vi "Parse PJVS Voltages.vi"(8 "error in":errorcluster, 11 "Data":string) -> (0 "error out":errorcluster, 3 "PJVS Voltages":T1={"DC Voltage (S)"=nan, "AC Josephson Voltage RMS (V)"=nan, "Number of steps"=-1, "AC Voltages (V)"=[]} {"AC Voltages (V)" format="%#_10g"; "AC Josephson Voltage RMS (V)" format="%#_10g"; "DC Voltage (S)" format="%#_10g"})   [LabVIEW 2019, in "ACSVcontrol-driver.lvlib"]
doc: "Parse data recieved from PJVS with PJVS voltages data."
uses:
  ACSVcontrol-driver.lvlib
  Public/Type Definitions/PJVS Voltages.ctl
  <vilib>/Utility/error.llb/Error Cluster From Error Code.vi
  <vilib>/ErrorRing/Error Ring.xnode
panel:
  out "Waveform Graph":dbl[](graph)
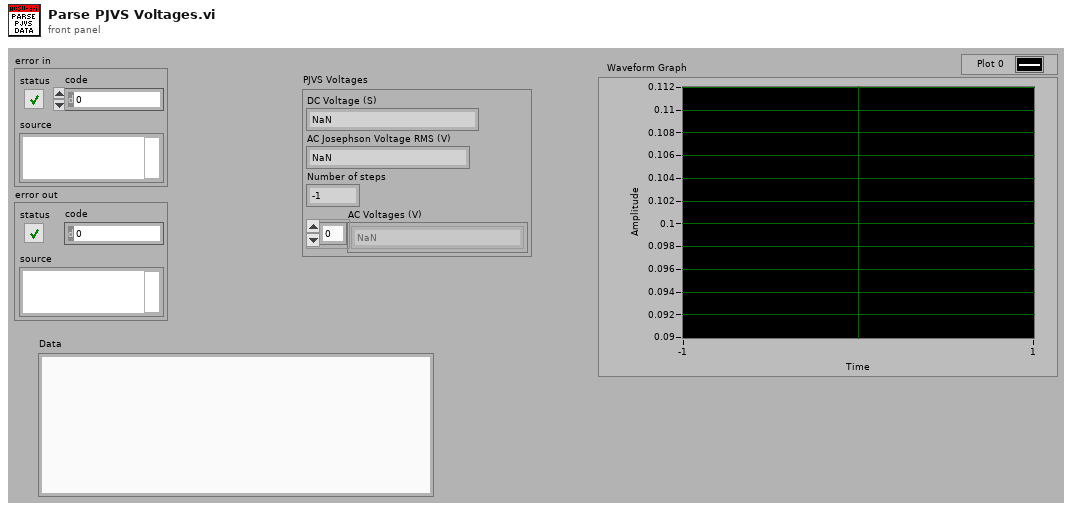
[diagram p1: front panel]
types:
  T1 = typedef "ACSVcontrol-driver.lvlib/PJVS Voltages.ctl" = cluster{"DC Voltage (S)":dbl, "AC Josephson Voltage RMS (V)":dbl, "Number of steps":i32, "AC Voltages (V)":dbl[]}
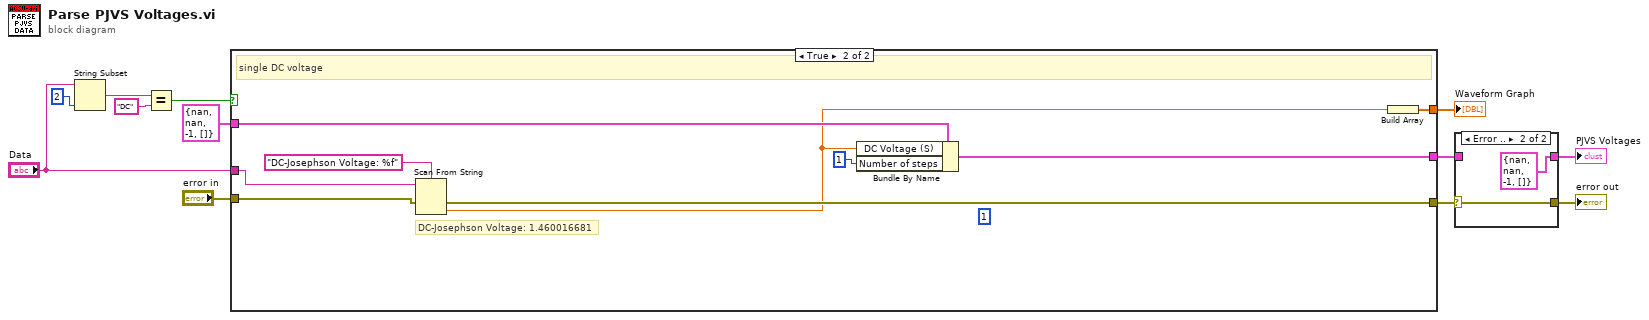
[diagram p0: block diagram]
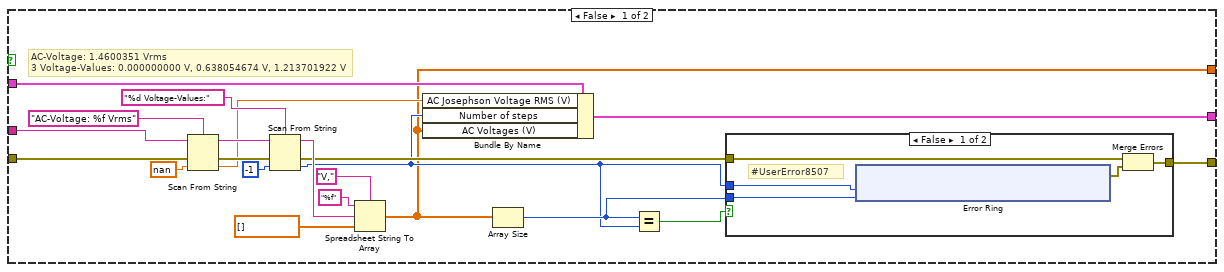
[diagram p3: hidden frame]
diagram:
  n1 = String Subset(string="Data", length (rest)=2 ("length (rest)")) -> (substring=w11:string)  [unwired: 1 in]
  n2 = Equal?(x=w11, y="DC") -> (x = y?=w9:bool)
  n3 = case shown="True" w9 {
    tunnel: "Data" -> [w32 w55]
    tunnel: "error in" -> [w21 w54]
    tunnel: [w20 w53] -> w6
    tunnel: T1 {"DC Voltage (S)"=nan, "AC Josephson Voltage RMS (V)"=nan, "Number of steps"=-1, "AC Voltages (V)"=[]} ("PJVS Voltages") -> [w14 w52]
    tunnel: [w15 w51] -> w2
    tunnel: [w13 w49] -> w1
    frame False {
      # "AC-Voltage: 1.4600351 Vrms\n3 Voltage-Values: 0.000000000 V, 0.638054674 V, 1.213701922 V"
      n4 = Scan From String(format string="AC-Voltage: %f Vrms", input string=w32, error in=w21, default 1=nan ("default value 1")) -> (remaining string=w30:string, error out=w25:errorcluster, output 1=w17:dbl)  [unwired: 1 in, 1 out]
      n5 = Scan From String(format string="%d Voltage-Values:", input string=w30, error in=w25, default 1=-1 ("default value 1")) -> (remaining string=w27:string, error out=w18:errorcluster, output 1=w16:i32)  [unwired: 1 in, 1 out]
      n6 = Spreadsheet String To Array(delimiter (Tab)="V,", format string="%f", spreadsheet string=w27, array type (2D Dbl)=dbl[] []) -> (array=w13:dbl[])
      n7 = Bundle By Name(cluster=w14, "AC Josephson Voltage RMS (V)"=w17, "Number of steps"=w16, "AC Voltages (V)"=w13) -> (w15:T1)
      n8 = Array Size(array=w13) -> (size(s)=w19:i32)
      n9 = Equal?(x=w19, y=w16) -> (x = y?=w22:bool)
      n10 = case shown="False" w22 {
        tunnel: [w34 w47] -> w20
        tunnel: w18 -> [w35 w47]
        tunnel: w16 -> [w38 _]
        tunnel: w19 -> [w37 _]
        frame False {
          # "#UserError8507"
          n11 = xnode "Error Ring"("parameter 0"=w38, "parameter 1"=w37) -> ("error out"=w36:errorcluster)
          n12 = Merge Errors(w35, w36) -> (w34:errorcluster)
        }
        frame True {
        }
      }
    }
    frame True {
      (unwired) 1 ("default value 1")
      # "DC-Josephson Voltage: 1.460016681"
      # "single DC voltage"
      n13 = Scan From String(format string="DC-Josephson Voltage: %f", input string=w55, error in=w54) -> (error out=w53:errorcluster, output 1=w48:dbl)  [unwired: 2 in, 2 out]
      n14 = Bundle By Name(cluster=w52, "DC Voltage (S)"=w48, "Number of steps"=1) -> (w51:T1)
      n15 = Build Array(w48) -> (w49:dbl[])
    }
  }
  "Waveform Graph" <- w1
  n16 = case shown="Error .." w6 {
    selector: w6 -> [w58 w60]
    tunnel: [w58 w60] -> w5
    tunnel: [w57 T1 {"DC Voltage (S)"=nan, "AC Josephson Voltage RMS (V)"=nan, "Number of steps"=-1, "AC Voltages (V)"=[]} ("PJVS Voltages")] -> w3
    tunnel: w2 -> [w57 _]
    frame No Error {
    }
    frame Error {
    }
  }
  "error out" <- w5
  "PJVS Voltages" <- w3
